vi "ExampleRestartableReader.vi"() -> ()   [LabVIEW 2011]
uses:
  Reader/readType.ctl
  0x2 Typedefs/RIO-OCU update controls.ctl
  2-Think/2 Typedefs/generalized sensor status.ctl
  2-Think/2 Typedefs/indicator LED.ctl
  2-Think/2 Typedefs/generalized actuator status.ctl
  2-Think/2 Typedefs/Which Boat.ctl
  2-Think/2 Typedefs/robot velocity.ctl
  2-Think/2 Typedefs/UTM Location.ctl
  2-Think/2 Typedefs/heading.ctl
  2-Think/2 Typedefs/rate of turn.ctl
  2-Think/2 Typedefs/pitch and roll.ctl
  2-Think/2 Typedefs/apparent wind.ctl
  2-Think/2 Typedefs/apparent wind speed.ctl
  2-Think/2 Typedefs/apparent wind direction.ctl
  2-Think/2 Typedefs/Velocity.ctl
  2-Think/2 Typedefs/absolute wind direction.ctl
  2-Think/2 Typedefs/absolute wind speed.ctl
  2-Think/2 Typedefs/absolute water current vector.ctl
  2-Think/2 Typedefs/rudder angle.ctl
  2-Think/2 Typedefs/sail setpt.ctl
  0x2 Typedefs/manual override.ctl
  2-Think/2 Typedefs/setpoints to boat.ctl
  0x2 Typedefs/Current Waypoint.ctl
  2-Think/2 Typedefs/Goodness Fns Indicator.ctl
  2-Think/2 Typedefs/UTM Circle.ctl
  2-Think/2 Globals/2 Global.vi
  Reader/NetworkStreamReader.lvclass
panel:
  out "error out 2":errorcluster
  out "Connected?":bool
  out "Iteration Time Stamp":timestamp
  out "OCU Time Stamp":timestamp
  in  "stop":bool
  out "Monitored Items from RIO":T1 {"Absolute Wind"."East" format="%#_5g"; "Robot Pitch/Roll"."Roll" format="%05.1f"; "Robot Pitch/Roll"."Pitch" format="%05.1f"; "Robot\nRate of Turn" format="%05.1f"; "Robot\nHeading" format="%05.1f"; "Robot UTM Location"."North" format="%#_10f"; "Robot UTM Location"."East" format="%#_8f"}
  in  "Read Type":T25=enum."Most current"
  in  "Loop delay (ms)":u32
  out "element":variant
  out "data":i32
  # "Note: writer is running at 50 ms"
  # "How Am I?"
  # "Where Am I?"
  # "Path Planning"
  # "From Planning Functions"
  # "(this is not a cluster because subitems\nare generated in parallel code)"
  # "What's Around Me?"
  # "As Measured"
  # "As Measured"
  # "Loop Rates"
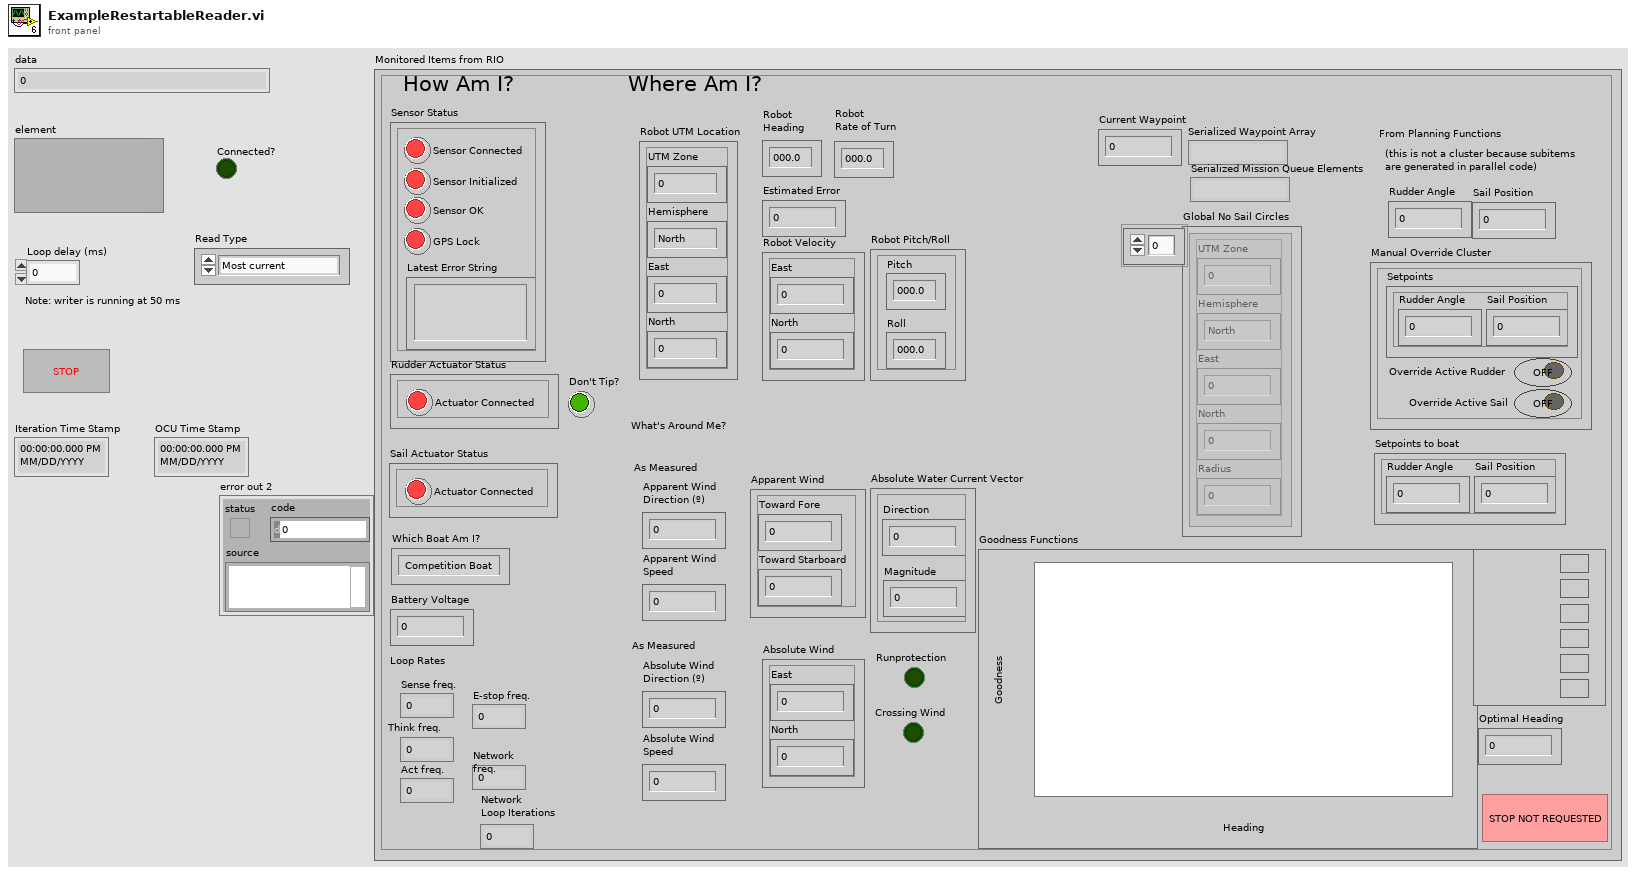
[diagram p1: front panel]
types:
  T1 = typedef "RIO-OCU update controls.ctl" = cluster{"Sensor Status":T2, "Battery Voltage":dbl, "Rudder Actuator Status":T4, "Sail Actuator Status":T4, "Which Boat Am I?":T5, "Robot Velocity":T6, "Robot UTM Location":T7, "Robot\nHeading ":T8, "Robot\nRate of Turn":T9, "Robot Pitch/Roll":T10, "Apparent Wind":T11, "Apparent Wind\nSpeed":T12, "Apparent Wind\nDirection (º)":T13, "Absolute Wind":T14, "Absolute Wind\nDirection (º)":T15, "Absolute Wind\nSpeed":T16, "Absolute Water Current Vector":T17, "Rudder Angle":T18, "Sail Position":T19, "Manual Override Cluster":T20, "Setpoints to boat":T21, "Current Waypoint":T22, "Think freq.":dbl, "Sense freq.":dbl, "Act freq.":dbl, "E-stop freq.":dbl, "Network \nfreq.":dbl, "Network \nLoop Iterations":i64, "E-Stop":bool, "Serialized Waypoint Array":string, "Serialized Mission Queue Elements":string, "Goodness Functions":T23, "Global No Sail Circles":T24[], "Runprotection":bool, "Optimal Heading":dbl, "Crossing Wind":bool, "Estimated Error":dbl, "Don't Tip?":bool}
  T2 = typedef "generalized sensor status.ctl" = cluster{"Sensor Connected":T3, "Sensor Initialized":T3, "Sensor OK":T3, "Latest Error String":string, "GPS Lock":T3}
  T3 = typedef "indicator LED.ctl" = bool
  T4 = typedef "generalized actuator status.ctl" = cluster{"Actuator Connected":T3}
  T5 = typedef "Which Boat.ctl" = enum16{"Competition Boat", "Small RC", "Simulation"}
  T6 = typedef "robot velocity.ctl" = cluster{"East":dbl, "North":dbl}
  T7 = typedef "UTM Location.ctl" = cluster{"UTM Zone":dbl, "Hemisphere":enum16{"North", "South"}, "East":dbl, "North":dbl}
  T8 = typedef "heading.ctl" = dbl
  T9 = typedef "rate of turn.ctl" = dbl
  T10 = typedef "pitch and roll.ctl" = cluster{"Pitch":dbl, "Roll":dbl}
  T11 = typedef "apparent wind.ctl" = cluster{"Toward Fore":dbl, "Toward Starboard":dbl}
  T12 = typedef "apparent wind speed.ctl" = dbl
  T13 = typedef "apparent wind direction.ctl" = dbl
  T14 = typedef "Velocity.ctl" = cluster{"East":dbl, "North":dbl}
  T15 = typedef "absolute wind direction.ctl" = dbl
  T16 = typedef "absolute wind speed.ctl" = dbl
  T17 = typedef "absolute water current vector.ctl" = cluster{"Direction":T13, "Magnitude":T13}
  T18 = typedef "rudder angle.ctl" = dbl
  T19 = typedef "sail setpt.ctl" = dbl
  T20 = typedef "manual override.ctl" = cluster{"Override Active Rudder":bool, "Setpoints":T21, "Override Active Sail":bool}
  T21 = typedef "setpoints to boat.ctl" = cluster{"Sail Position":T19, "Rudder Angle":T18}
  T22 = typedef "Current Waypoint.ctl" = i32
  T23 = typedef "Goodness Fns Indicator.ctl" = cluster{dbl, dbl, dbl[][]}
  T24 = typedef "UTM Circle.ctl" = cluster{"UTM Zone":dbl, "Hemisphere":enum16{"North", "South"}, "East":dbl, "North":dbl, "Radius":dbl}
  T25 = typedef "NetworkStreamReader.lvclass/readType.ctl" = enum16{"Next in buffer", "Most current"}
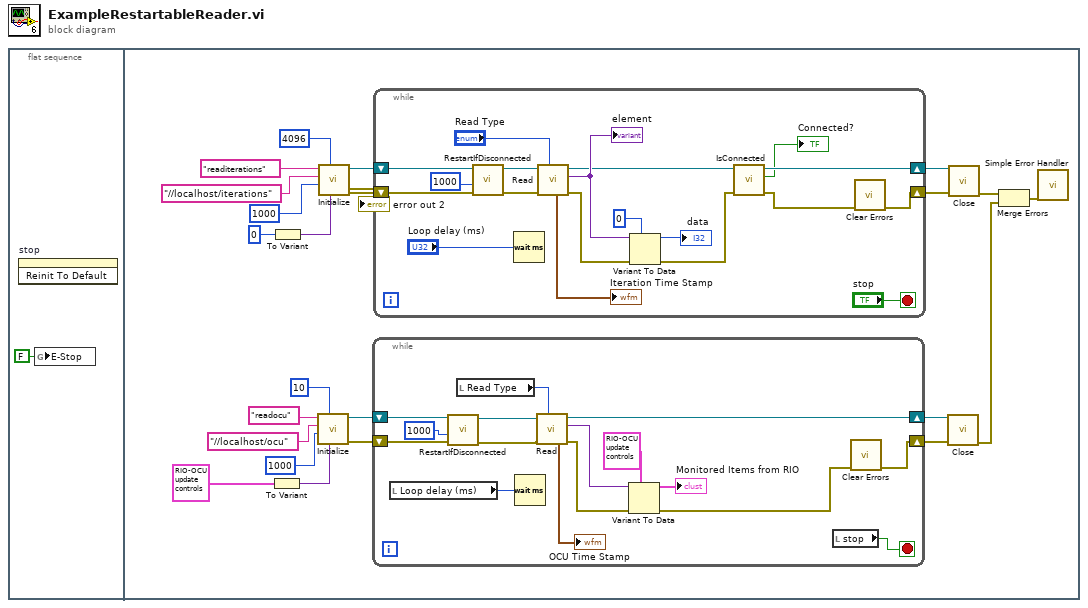
[diagram p0: block diagram]
diagram:
  n1 = flat-sequence {
    frame #0 {
      n2 = invoke on="stop" class="Bool (strict)" method="Reinit To Default"() -> ()  [unwired: 3 in, 3 out]
      n3 = global write "2 Global.vi" "E-Stop"(FALSE ("E-Stop")) -> ()
    }
    frame #1 {
      n4 = To Variant(anything=T1 {"Sensor Status"={"Sensor Connected"=FALSE, "Sensor Initialized"=FALSE, "Sensor OK"=FALSE, "Latest Error String"="", "GPS Lock"=FALSE}, "Battery Voltage"=0.0, "Rudder Actuator Status"={"Actuator Connected"=FALSE}, "Sail Actuator Status"={"Actuator Connected"=FALSE}, "Which Boat Am I?"=enum."Competition Boat", "Robot Velocity"={"East"=0.0, "North"=0.0}, "Robot UTM Location"={"UTM Zone"=0.0, "Hemisphere"=enum."North", "East"=0.0, "North"=0.0}, "Robot\nHeading "=0.0, "Robot\nRate of Turn"=0.0, "Robot Pitch/Roll"={"Pitch"=0.0, "Roll"=0.0}, "Apparent Wind"={"Toward Fore"=0.0, "Toward Starboard"=0.0}, "Apparent Wind\nSpeed"=0.0, "Apparent Wind\nDirection (º)"=0.0, "Absolute Wind"={"East"=0.0, "North"=0.0}, "Absolute Wind\nDirection (º)"=0.0, "Absolute Wind\nSpeed"=0.0, "Absolute Water Current Vector"={"Direction"=0.0, "Magnitude"=0.0}, "Rudder Angle"=0.0, "Sail Position"=0.0, "Manual Override Cluster"={"Override Active Rudder"=FALSE, "Setpoints"={"Sail Position"=0.0, "Rudder Angle"=0.0}, "Override Active Sail"=FALSE}, "Setpoints to boat"={"Sail Position"=0.0, "Rudder Angle"=0.0}, "Current Waypoint"=0, "Think freq."=0.0, "Sense freq."=0.0, "Act freq."=0.0, "E-stop freq."=0.0, "Network \nfreq."=0.0, "Network \nLoop Iterations"=0, "E-Stop"=FALSE, "Serialized Waypoint Array"="", "Serialized Mission Queue Elements"="", "Goodness Functions"={0.0, 0.0, []}, "Global No Sail Circles"=[], "Runprotection"=FALSE, "Optimal Heading"=0.0, "Crossing Wind"=FALSE, "Estimated Error"=0.0, "Don't Tip?"=FALSE} ("Monitored Items from RIO")) -> (Variant=w18:variant)
      n5 = To Variant(anything=0) -> (Variant=w19:variant)
      n6 = call "Initialize.vi"("Default return"=w18, "reader buffer size"=10 ("writer buffer size"), "connection timeout"=1000, "writer url"="//localhost/ocu", "reader name"="readocu") -> ("error out"=w13:errorcluster, "NetworkStreamWriter out"=w15:refnum<class "NetworkStreamReader.lvclass">)  [unwired: 3 in, 2 out]
      n7 = call "Initialize.vi"("Default return"=w19, "reader buffer size"=4096 ("writer buffer size"), "connection timeout"=1000, "writer url"="//localhost/iterations", "reader name"="readiterations") -> ("error out"=w25:errorcluster, "NetworkStreamWriter out"=w23:refnum<class "NetworkStreamReader.lvclass">, "error out 2"=→"error out 2":errorcluster)  [unwired: 3 in, 1 out]
      n8 = while {
        shift-right: [w27] -> w17
        shift-left: w15 -> [w31]
        shift-right: [w32] -> w16
        shift-left: w13 -> [w30]
        stop <- w35 stop-if-true
        n9 = local read "Loop delay (ms)"() -> (w39:u32)
        n10 = call "RestartIfDisconnected.vi"("error in (no error)"=w30, "connection timeout"=1000, "NetworkStreamReader in"=w31) -> ("error out"=w28:errorcluster, "NetworkStreamReader out"=w29:refnum<class "NetworkStreamReader.lvclass">)  [unwired: 7 in]
        n11 = local read "Read Type"() -> (w40:T25)
        n12 = Wait (ms)(milliseconds to wait=w39) -> ()  [unwired: 1 out]
        n13 = call "Read.vi"("Read Type"=w40, "error in (no error)"=w28, "NetworkStreamReader in"=w29) -> ("error out"=w38:errorcluster, "element"=w41:variant, "NetworkStreamReader out"=w27:refnum<class "NetworkStreamReader.lvclass">, "Time Stamp"=→"OCU Time Stamp":timestamp)  [unwired: 4 in, 1 out]
        n14 = Variant To Data(error in=w38, type=T1 {"Sensor Status"={"Sensor Connected"=FALSE, "Sensor Initialized"=FALSE, "Sensor OK"=FALSE, "Latest Error String"="", "GPS Lock"=FALSE}, "Battery Voltage"=0.0, "Rudder Actuator Status"={"Actuator Connected"=FALSE}, "Sail Actuator Status"={"Actuator Connected"=FALSE}, "Which Boat Am I?"=enum."Competition Boat", "Robot Velocity"={"East"=0.0, "North"=0.0}, "Robot UTM Location"={"UTM Zone"=0.0, "Hemisphere"=enum."North", "East"=0.0, "North"=0.0}, "Robot\nHeading "=0.0, "Robot\nRate of Turn"=0.0, "Robot Pitch/Roll"={"Pitch"=0.0, "Roll"=0.0}, "Apparent Wind"={"Toward Fore"=0.0, "Toward Starboard"=0.0}, "Apparent Wind\nSpeed"=0.0, "Apparent Wind\nDirection (º)"=0.0, "Absolute Wind"={"East"=0.0, "North"=0.0}, "Absolute Wind\nDirection (º)"=0.0, "Absolute Wind\nSpeed"=0.0, "Absolute Water Current Vector"={"Direction"=0.0, "Magnitude"=0.0}, "Rudder Angle"=0.0, "Sail Position"=0.0, "Manual Override Cluster"={"Override Active Rudder"=FALSE, "Setpoints"={"Sail Position"=0.0, "Rudder Angle"=0.0}, "Override Active Sail"=FALSE}, "Setpoints to boat"={"Sail Position"=0.0, "Rudder Angle"=0.0}, "Current Waypoint"=0, "Think freq."=0.0, "Sense freq."=0.0, "Act freq."=0.0, "E-stop freq."=0.0, "Network \nfreq."=0.0, "Network \nLoop Iterations"=0, "E-Stop"=FALSE, "Serialized Waypoint Array"="", "Serialized Mission Queue Elements"="", "Goodness Functions"={0.0, 0.0, []}, "Global No Sail Circles"=[], "Runprotection"=FALSE, "Optimal Heading"=0.0, "Crossing Wind"=FALSE, "Estimated Error"=0.0, "Don't Tip?"=FALSE} ("Monitored Items from RIO"), Variant=w41) -> (data=→"Monitored Items from RIO":T1, error out=w26:errorcluster)
        n15 = local read "stop"() -> (w35:bool)
        n16 = call <vilib>:"Clear Errors.vi"("error in (no error)"=w26) -> ("error out"=w32:errorcluster)  [unwired: 6 in]
      }
      n17 = while {
        shift-right: [w46] -> w21
        shift-left: w23 -> [w49]
        shift-right: [w52] -> w22
        shift-left: w25 -> [w48]
        stop <- "stop" stop-if-true
        n18 = call "RestartIfDisconnected.vi"("error in (no error)"=w48, "connection timeout"=1000, "NetworkStreamReader in"=w49) -> ("error out"=w50:errorcluster, "NetworkStreamReader out"=w51:refnum<class "NetworkStreamReader.lvclass">)  [unwired: 7 in]
        n19 = Wait (ms)(milliseconds to wait="Loop delay (ms)") -> ()  [unwired: 1 out]
        n20 = call "Read.vi"("Read Type"="Read Type", "error in (no error)"=w50, "NetworkStreamReader in"=w51) -> ("error out"=w55:errorcluster, "element"=w60:variant, "NetworkStreamReader out"=w47:refnum<class "NetworkStreamReader.lvclass">, "Time Stamp"=→"Iteration Time Stamp":timestamp)  [unwired: 4 in, 1 out]
        "element" <- w60
        n21 = Variant To Data(error in=w55, type=0, Variant=w60) -> (data=→"data":i32, error out=w45:errorcluster)
        n22 = call "IsConnected.vi"("error in (no error)"=w45, "NetworkStreamReader in"=w47) -> ("error out"=w44:errorcluster, "Connected?"=→"Connected?":bool, "NetworkStreamReader out"=w46:refnum<class "NetworkStreamReader.lvclass">)  [unwired: 7 in]
        n23 = call <vilib>:"Clear Errors.vi"("error in (no error)"=w44) -> ("error out"=w52:errorcluster)  [unwired: 6 in]
      }
      n24 = call "Close.vi"("error in (no error)"=w16, "NetworkStreamReader in"=w17) -> ("error out"=w11:errorcluster)  [unwired: 8 in, 1 out]
      n25 = call "Close.vi"("error in (no error)"=w22, "NetworkStreamReader in"=w21) -> ("error out"=w12:errorcluster)  [unwired: 8 in, 1 out]
      n26 = Merge Errors(w12, w11) -> (w10:errorcluster)
      n27 = call <vilib>:"Simple Error Handler.vi"("error in (no error)"=w10) -> ()  [unwired: 4 in, 5 out]
    }
  }
